vi "New Stream To Disk Transport.vi"(9 "Channel Name":string, 10 "File Path":path) -> (0 "error out":errorcluster, 3 "StreamToDisk Out":refnum<class "StreamToDisk.lvclass">)   [LabVIEW 2015, in "Transport.lvlib" / "StreamToDisk.lvclass"]
doc: "<License>\nCopyright © 2017 Composed Systems, LLC | All rights reserved\nwww.composed.io\n\nAuthor: Ethan Stern <ethan.stern@composed.io>\n\nThis software is provided \"AS IS\" WITHOUT WARRANTIES, either express or implied, AND IS FOR EDUCATIONAL PURPOSES ONLY.\n</License>"
uses:
  StreamToDisk.lvclass
  StreamToDisk.lvclass/StreamToDisk.ctl
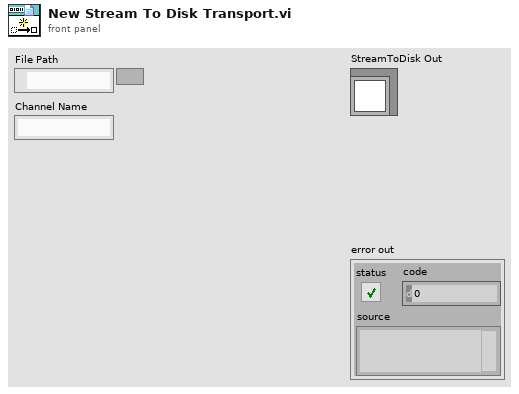
[diagram p1: front panel]
types:
  T1 = enum16{"open", "open or create", "create or replace", "create", "open (read-only)"}
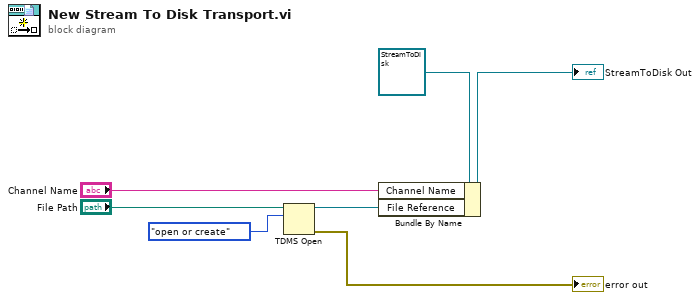
[diagram p0: block diagram]
diagram:
  n1 = TDMS Open(10:T1."open or create" ("operation (0:open)"), 11:"File Path") -> (0:→"error out":errorcluster, 3:w3:refnum<k34>)  [unwired: 5 in]
  n2 = Bundle By Name(cluster=refnum<class "StreamToDisk.lvclass"> refnum ("TerminalReference in"), "Channel Name"="Channel Name", "File Reference"=w3) -> (→"StreamToDisk Out":refnum<class "StreamToDisk.lvclass">)
